vi "Property Node Demo.vi"() -> ()   [LabVIEW 2017]
panel:
  in  "offset":dbl(knob) scale=0.0..10.0
  in  "gain":dbl(knob) scale=0.0..10.0
  in  "show/hide \nadvanced control":bool
  in  "on/off":bool
  out "Tension (kN)":dbl(knob) scale=0.0..10.0
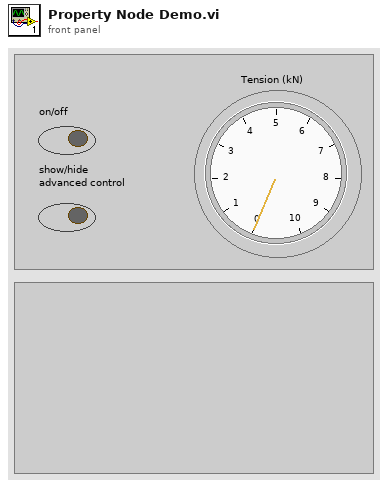
[diagram p1: front panel]
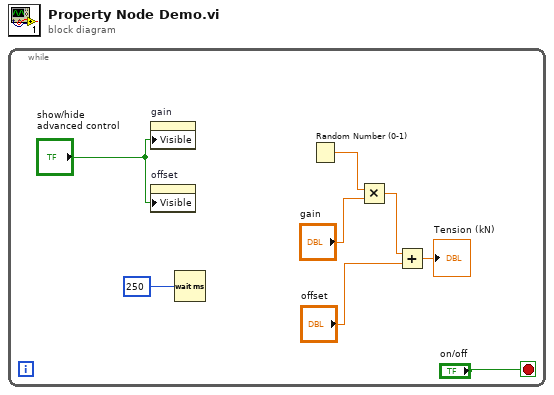
[diagram p0: block diagram]
diagram:
  n1 = while {
    stop <- "on/off" stop-if-true
    n2 = property on="gain" class="Knob (strict)"("Visible"="show/hide \nadvanced control") -> ()  [unwired: 2 in, 2 out]
    n3 = property on="offset" class="Knob (strict)"("Visible"="show/hide \nadvanced control") -> ()  [unwired: 2 in, 2 out]
    n4 = Wait (ms)(milliseconds to wait=250) -> ()  [unwired: 1 out]
    n5 = Random Number (0-1)() -> (number: 0 to 1=w7:dbl)
    n6 = Multiply(x=w7, y="gain") -> (x*y=w4:dbl)
    n7 = Add(x=w4, y="offset") -> (x+y=→"Tension (kN)":dbl)
  }
